vi "Factorial.vi"(1 "Input_num":i32) -> (0 "Numeric":i32)   [LabVIEW 2015]
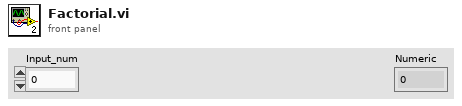
[diagram p1: front panel]
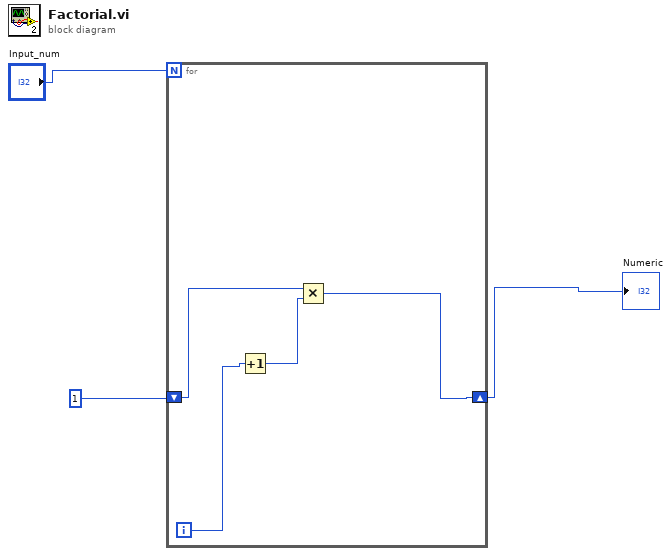
[diagram p0: block diagram]
diagram:
  n1 = for {
    N: "Input_num" -> [_]
    shift-right: [w4] -> w3
    shift-left: 1 -> [w5]
    i -> [w7]
    n2 = Increment(x=w7) -> (x+1=w6:i32)
    n3 = Multiply(x=w5, y=w6) -> (x*y=w4:i32)
  }
  "Numeric" <- w3
